vi "Check Buffer Client.vi"(8 "error in":errorcluster, 11 "gRPC ID in":T1) -> (0 "error out":errorcluster, 2 "Payload":u8[](array[numeric]), 3 "gRPC ID out":T1)   [LabVIEW 2025, in "CAN-LIN Raw Bus Capture UI.lvlib"]
uses:
  CAN-LIN Raw Bus Capture UI.lvlib
  OOB gRPC Client/OOB gRPC Client.lvlib
  OOB gRPC Client/RPC Messages/hwval_GenericRequest.ctl
  <vilib>/gRPC/LabVIEW gRPC Library/Shared/grpcId.ctl
  <vilib>/gRPC/LabVIEW gRPC Library/grpc-lvsupport-release.lvlib
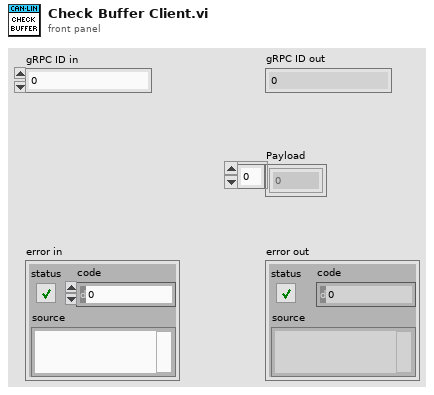
[diagram p1: front panel]
types:
  T1 = typedef "grpc-lvsupport-release.lvlib/grpcId.ctl" = u64
  T2 = typedef "OOB gRPC Client.lvlib/hwval_GenericRequest.ctl" = cluster{"Command":string, "Payload":u8[]}
  T3 = typedef "OOB gRPC Client.lvlib/hwval_GenericResponse.ctl" = cluster{"Payload":u8[]}
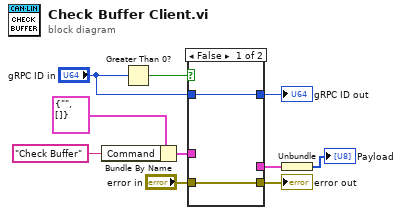
[diagram p0: block diagram]
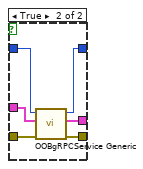
[diagram p2: hidden frame]
diagram:
  n1 = Bundle By Name(cluster=T2 {"Command"="", "Payload"=[]} ("Request Data"), "Command"="Check Buffer") -> (w4:T2)
  n2 = Greater Than 0?(x="gRPC ID in") -> (x > 0?=w2:bool)
  n3 = case shown="False" w2 {
    tunnel: [_ w18] -> w6
    tunnel: w4 -> [_ w17]
    tunnel: [w12 w16] -> w8
    tunnel: "error in" -> [w12 w15]
    tunnel: "gRPC ID in" -> [w11 w14]
    tunnel: [w11 w13] -> w1
    frame False {
    }
    frame True {
      n4 = call "OOBgRPCService Generic.vi"("error in"=w15, "Request Data"=w17, "gRPC ID"=w14) -> ("error out"=w16:errorcluster, "Response Data"=w18:T3, "gRPC ID out"=w13:T1)  [unwired: 6 in]
    }
  }
  "error out" <- w8
  "gRPC ID out" <- w1
  n5 = Unbundle(w6) -> ("Payload"=→"Payload":u8[])
